vi "Configure Pulse Width.vi"(6 "Reference Value (50%)":dbl=50.0 format="%#_4g", 8 "error in (no error)":errorcluster, 9 "Reference Type (0:Percent)":i32(ring) items=["Percent", "Voltage"], 10 "Pulse Width Type (0:Positive)":i32(ring) items=["Positive", "Negative"], 11 "VISA resource name":refnum<visa-resource-name>) -> (0 "error out":errorcluster, 3 "VISA resource name out":refnum<visa-resource-name>)   [LabVIEW 2020, in "Counter.lvlib" / "PICOTEST U62XXA series.lvlib"]
doc: "Configure the Settings required for Pulse Width Measurements. Pulse Width Measurements can only be taken at channel 1.\n\n<B>Note:</B>\nThe U6220A model <B>does not</B> support the \"Pulse Width\" commands.\n\nThe measurement arming is coupled to Auto. Arming can be changed by calling any of the Arming VIs."
uses:
  PICOTEST U62XXA series.lvlib
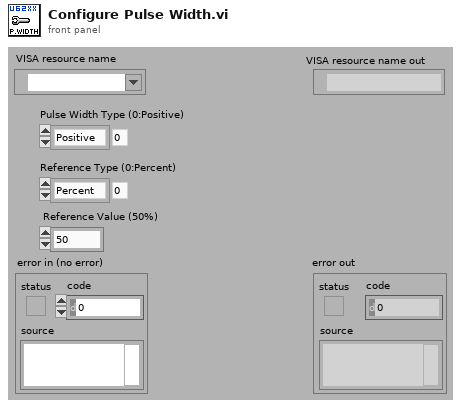
[diagram p1: front panel]
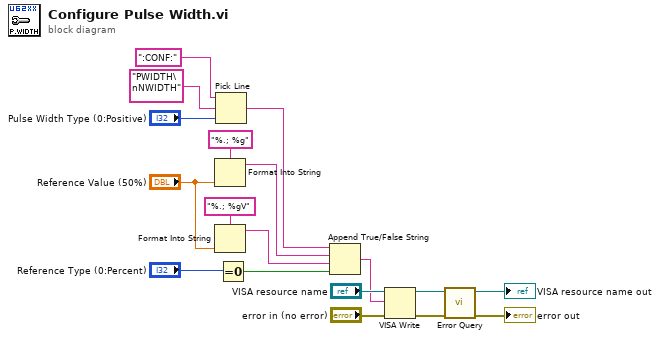
[diagram p0: block diagram]
diagram:
  n1 = Format Into String(format string="%.; %g", "Reference Value (50%)") -> (resulting string=w9:string)  [unwired: 2 in, 1 out]
  n2 = Format Into String(format string="%.; %gV", "Reference Value (50%)") -> (resulting string=w8:string)  [unwired: 2 in, 1 out]
  n3 = Pick Line(string ("")=":CONF:", multi-line string="PWIDTH\nNWIDTH", line index="Pulse Width Type (0:Positive)") -> (output string=w7:string)
  n4 = Equal To 0?(x="Reference Type (0:Percent)") -> (x = 0?=w10:bool)
  n5 = Append True/False String(1:w10, 2:w8, 3:w9, 4:w7) -> (0:w6:string)
  n6 = VISA Write(VISA resource name="VISA resource name", write buffer=w6, error in (no error)="error in (no error)") -> (VISA resource name out=w5:refnum<visa-resource-name>, error out=w3:errorcluster)  [unwired: 1 out]
  n7 = call "Error Query.vi"("error in (no error)"=w3, "VISA resource name"=w5) -> ("error out"=→"error out":errorcluster, "VISA resource name out"=→"VISA resource name out":refnum<visa-resource-name>)  [unwired: 6 in, 2 out]
